vi "Table-GetTblDataToUpdate.vi"(5 "OldVal":string[][](array[string]), 7 "NewVal":string[][](array[string]), 8 "error in (no error)":errorcluster, 11 "ERP-SpecificationManager in":refnum<class "ERP-SpecificationManager.lvclass">) -> (0 "error out":errorcluster, 3 "ERP-SpecificationManager out":refnum<class "ERP-SpecificationManager.lvclass">)   [LabVIEW 2013, in "ERP-SpecificationManager.lvclass"]
uses:
  ERP-SpecificationManager.lvclass
  ERP-SpecificationManager.lvclass/ERP-SpecificationManager.ctl
  <userlib>/_OpenG.lib/array/array.llb/Search 1D Array (Boolean)__ogtk.vi
  <userlib>/_OpenG.lib/array/array.llb/Empty 1D Array (I32)__ogtk.vi
panel:
  out "Index Chosen to Update":cluster{"Column":i32, "Row":i32}
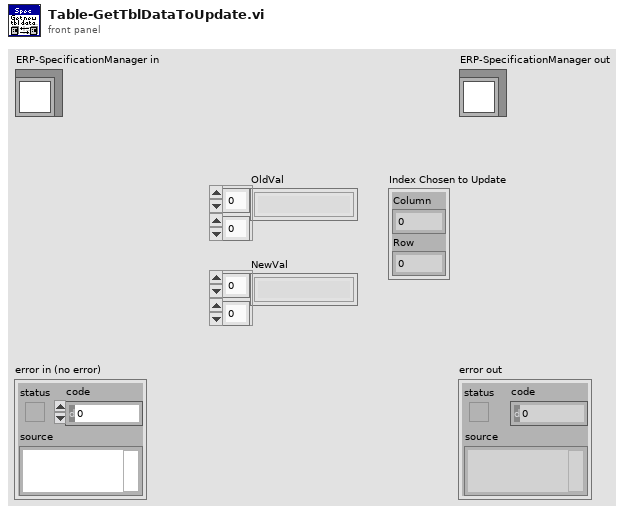
[diagram p1: front panel]
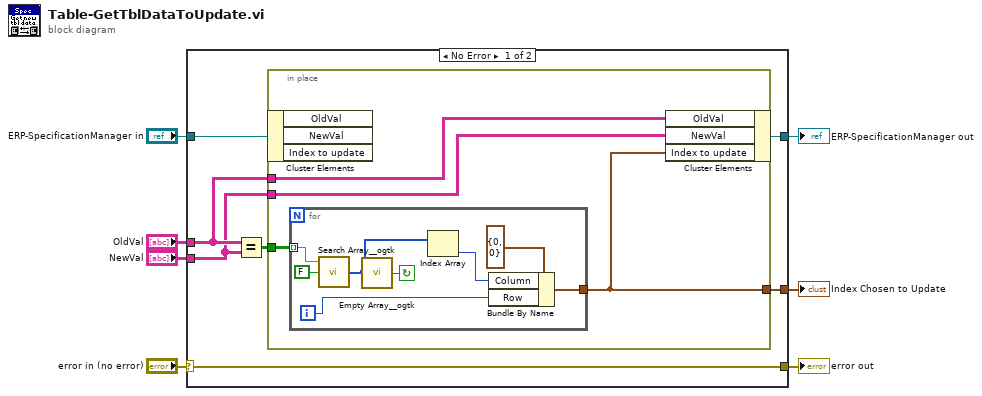
[diagram p0: block diagram]
diagram:
  n1 = case shown="No Error" "error in (no error)" {
    selector: "error in (no error)" -> [w14 w28]
    tunnel: [w14 w28] -> w6
    tunnel: [w9 w27] -> w4
    tunnel: "ERP-SpecificationManager in" -> [w10 w27]
    tunnel: "OldVal" -> [w12 _]
    tunnel: "NewVal" -> [w11 _]
    tunnel: [w8 _] -> w1
    frame No Error {
      n2 = Equal?(x=w12, y=w11) -> (x = y?=w13:bool[][])
      n3 = in-place {
        in-place-border: w13 -> [w18]
        in-place-border: w11 -> [w17]
        in-place-border: w12 -> [w16]
        in-place-border: [w15] -> w8
        n4 = in-place-cluster #1(w10) -> ()  [unwired: 3 out]
        n5 = for {
          tunnel: w18 -> [w26] mode=indexing
          tunnel: [w19] -> w15
          i -> [w20]
          stop <- w24 continue-if-true
          n6 = call-poly <userlib>:"Search Array__ogtk.vi"("Array"=w26, "Element Data"=FALSE) -> ("Indices of Elements"=w23:i32[])  [unwired: 7 in]
          n7 = call-poly <userlib>:"Empty Array__ogtk.vi"("Array"=w23) -> ("Empty Array?"=w24:bool)  [unwired: 8 in]
          n8 = Index Array(array=w23) -> (element=w21:i32)  [unwired: 1 in]
          n9 = Bundle By Name(cluster=cluster{"Column":i32, "Row":i32} {"Column"=0, "Row"=0}, "Column"=w21, "Row"=w20) -> (w19:cluster{"Column":i32, "Row":i32})
        }
        n10 = in-place-cluster #1("OldVal"=w16, "NewVal"=w17, "Index to update"=w15) -> (w9:refnum<class "ERP-SpecificationManager.lvclass">)
      }
    }
    frame Error {
    }
  }
  "error out" <- w6
  "ERP-SpecificationManager out" <- w4
  "Index Chosen to Update" <- w1
